vi "ScaleSquat_Angle.vi"(8 "ArmLength":cluster{"Upper":dbl, "Lower":dbl}, 9 "ScalingCoef Knee (1)":dbl=1.0, 10 "ScalingCoef Hip (1)":dbl=1.0, 11 "AverageJointAngles":dbl[][](array[numeric])) -> (1 "ScaledJointAngles":dbl[][](array[numeric]), 2 "ScaledGait":dbl[][](array[numeric]))   [LabVIEW 2016]
uses:
  <vilib>/Analysis/baseanly.llb/Real A x B.vi
  <vilib>/imath/engines/lvmath2/RunTimeEngine/NodeEndStatement/NIMS_NodeEndStatement_Output.vi
  <instcachedir>/0/NIMS_NodeEndStatement_Output_53EC0D466D134D7ABD903AC30B43404B.lvgen/NIMS_NodeEndStatement_Output_53EC0D466D134D7ABD903AC30B43404B_002.vi
  <vilib>/imath/engines/lvmath2/RunTimeEngine/ErrorHandling/NIMS_Finalize Error.vi
  <vilib>/Analysis/NI_AALBase.lvlib
panel:
  out "Waveform Graph 2":dbl[][](graph)
  out "JointAngles":dbl[][](graph)
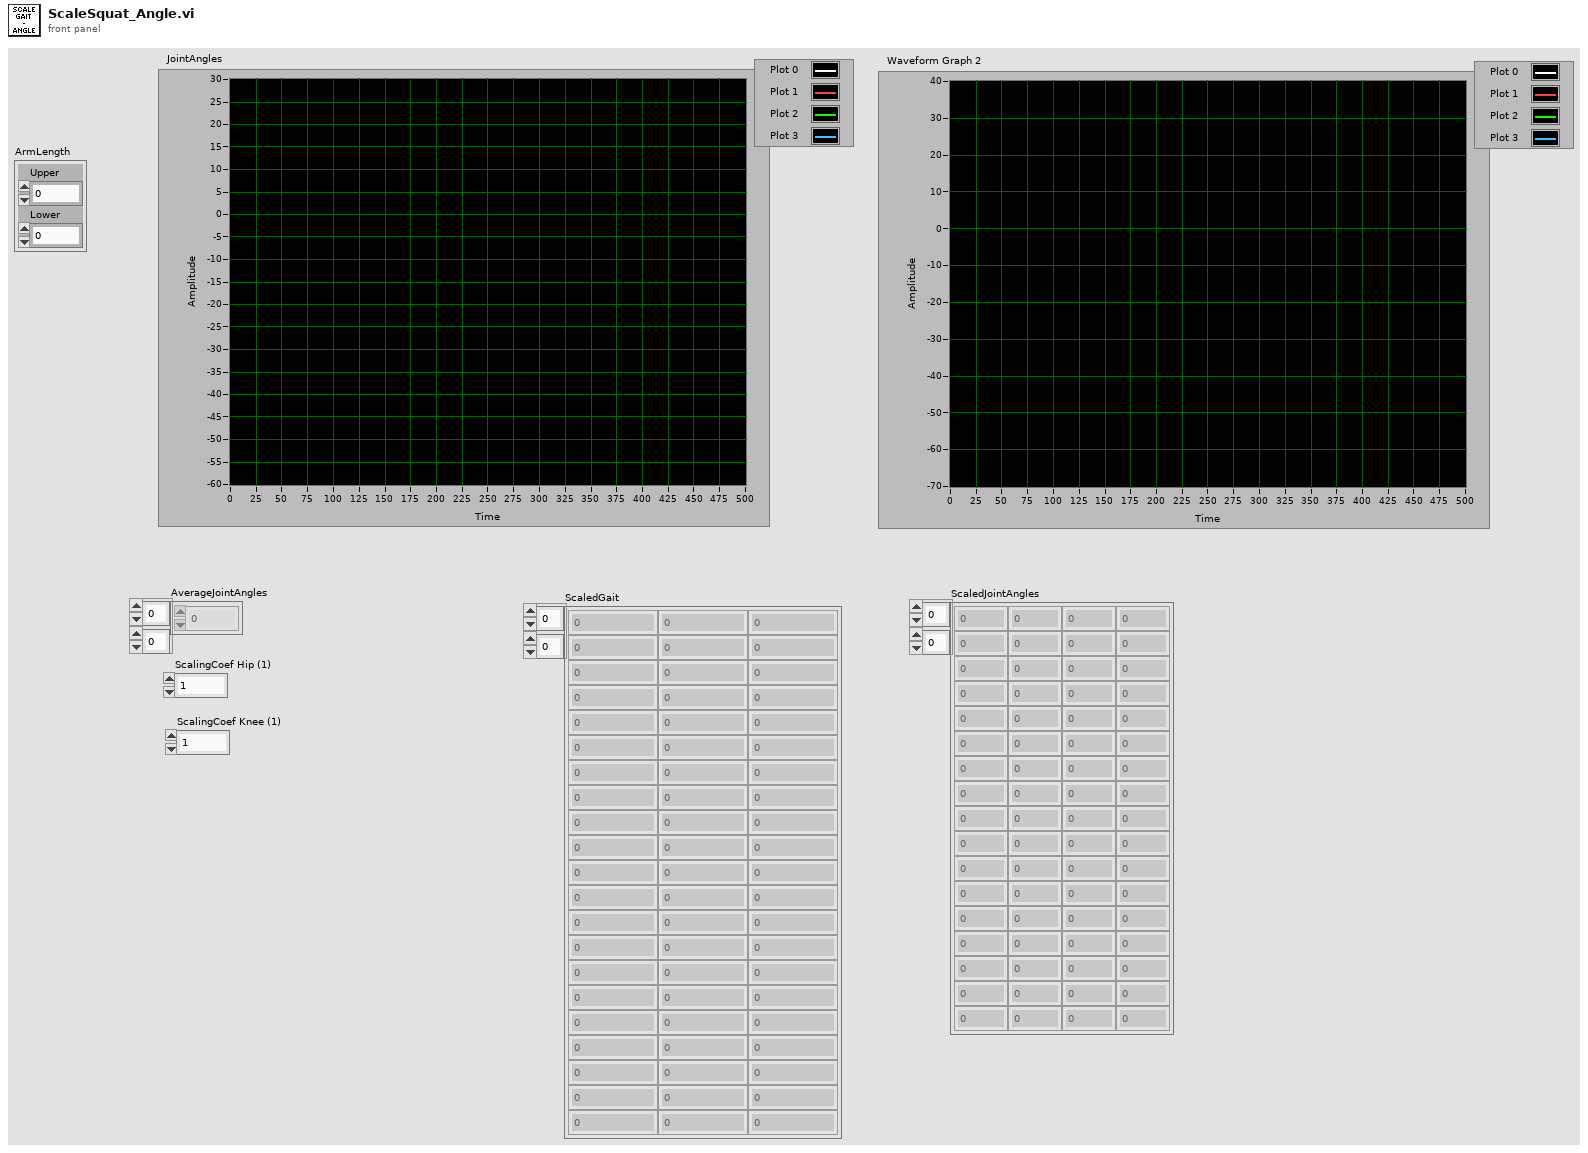
[diagram p1: front panel]
types:
  T1 = typedef "NI_Matrix.lvlib/RealMatrix.ctl" = dbl[][]
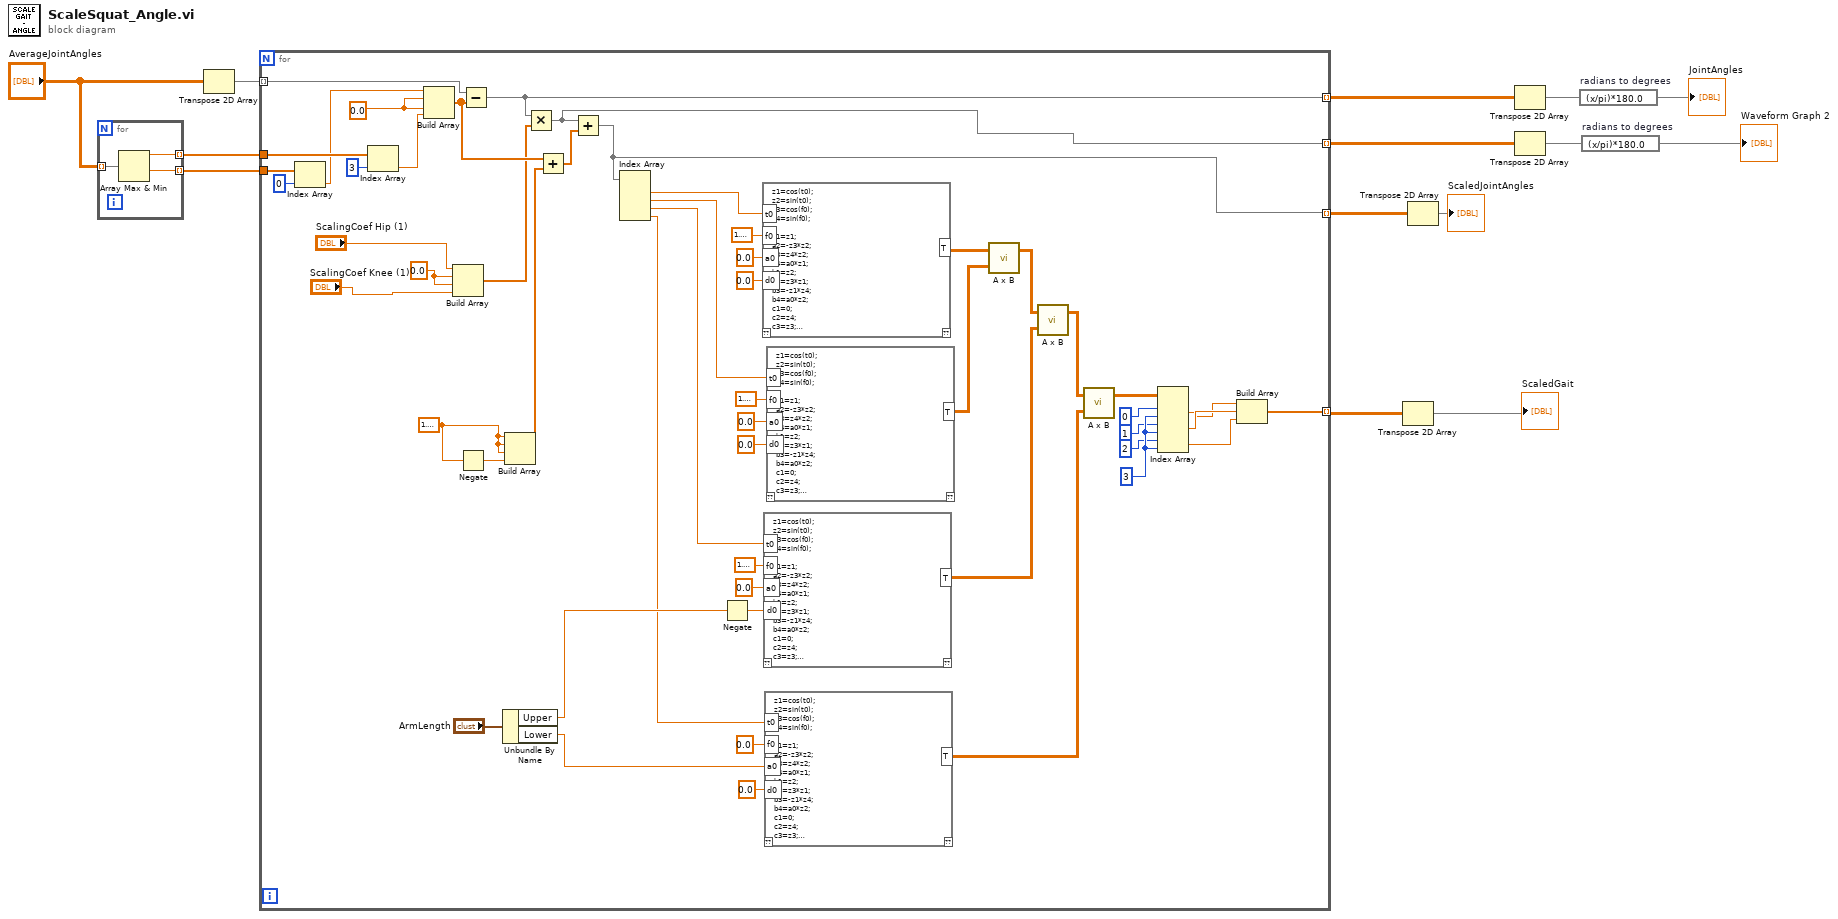
[diagram p0: block diagram]
diagram:
  n1 = for {
    tunnel: "AverageJointAngles" -> [w17] mode=indexing
    tunnel: [w16] -> w9 mode=indexing
    tunnel: [w15] -> w7 mode=indexing
    n2 = Array Max & Min(array=w17) -> (max value=w15:dbl, min value=w16:dbl)  [unwired: 2 out]
  }
  n3 = Transpose 2D Array(2D array="AverageJointAngles") -> (transposed array=w12:dbl[][])
  n4 = for {
    tunnel: w12 -> [w70] mode=indexing
    tunnel: [w65] -> w13 mode=indexing
    tunnel: w9 -> [w67]
    tunnel: [w29] -> w8 mode=indexing
    tunnel: w7 -> [w69]
    tunnel: [w41] -> w4 mode=indexing
    tunnel: [w28] -> w2 mode=indexing
    w19 = 0.0 ("element")
    w27 = 0.0 ("element")
    w22 = 1.5707963267948966
    w40 = 3 ("index (row)")
    n5 = Index Array(array=w67, index=0) -> (element=w66:dbl)
    n6 = Index Array(array=w69, index=3) -> (element=w30:dbl)
    n7 = Build Array(w66, w27, w27, w30) -> (w26:dbl[])
    n8 = Build Array("ScalingCoef Hip (1)", w19, w19, "ScalingCoef Knee (1)") -> (w21:dbl[])
    n9 = Negate(x=w22) -> (-x=w23:dbl)
    n10 = Subtract(x=w70, y=w26) -> (x-y=w65:dbl[])
    n11 = Unbundle By Name("ArmLength") -> ("Upper"=w35:dbl, "Lower"=w34:dbl)
    n12 = Build Array(w22, w22, w22, w23) -> (w24:dbl[])
    n13 = Multiply(x=w65, y=w21) -> (x*y=w29:dbl[])
    n14 = Add(x=w26, y=w24) -> (x+y=w25:dbl[])
    n15 = Add(x=w29, y=w25) -> (x+y=w28:dbl[])
    n16 = Index Array(array=w28) -> (element #1=w33:dbl, element #2=w60:dbl, element #3=w59:dbl, element #4=w32:dbl)  [unwired: 4 in]
    n17 = Negate(x=w35) -> (-x=w53:dbl)
    n18 = mathscript code="z1=cos(t0);\nz2=sin(t0);\nz3=cos(f0);\nz4=sin(f0);\n\na1=z1;\na2=-z3*z2;\na3=z4*z2;\na4=a0*z1;\nb1=z2;\nb2=z3*z1;\nb3=-z1*z4;\nb4=a0*z2;\nc1=0;\nc2=z4;\nc3=z3;\nc4=d0;\nd1=0;\nd2=0;\nd3=0;\nd4=1;\n\nT=[a1,a2,a3,a4;b1,b2,b3,b4;c1,c2,c3,c4;d1,d2,d3,d4];"("t0"=w33, "f0"=1.5707963267948966, "a0"=0.0, "d0"=0.0) -> ("T"=w51:dbl[][])  [unwired: 1 in, 1 out]
    n19 = mathscript code="z1=cos(t0);\nz2=sin(t0);\nz3=cos(f0);\nz4=sin(f0);\n\na1=z1;\na2=-z3*z2;\na3=z4*z2;\na4=a0*z1;\nb1=z2;\nb2=z3*z1;\nb3=-z1*z4;\nb4=a0*z2;\nc1=0;\nc2=z4;\nc3=z3;\nc4=d0;\nd1=0;\nd2=0;\nd3=0;\nd4=1;\n\nT=[a1,a2,a3,a4;b1,b2,b3,b4;c1,c2,c3,c4;d1,d2,d3,d4];"("t0"=w59, "f0"=1.5707963267948966, "a0"=0.0, "d0"=w53) -> ("T"=w48:dbl[][])  [unwired: 1 in, 1 out]
    n20 = mathscript code="z1=cos(t0);\nz2=sin(t0);\nz3=cos(f0);\nz4=sin(f0);\n\na1=z1;\na2=-z3*z2;\na3=z4*z2;\na4=a0*z1;\nb1=z2;\nb2=z3*z1;\nb3=-z1*z4;\nb4=a0*z2;\nc1=0;\nc2=z4;\nc3=z3;\nc4=d0;\nd1=0;\nd2=0;\nd3=0;\nd4=1;\n\nT=[a1,a2,a3,a4;b1,b2,b3,b4;c1,c2,c3,c4;d1,d2,d3,d4];"("t0"=w32, "f0"=0.0 ("a0"), "a0"=w34, "d0"=0.0) -> ("T"=w46:dbl[][])  [unwired: 1 in, 1 out]
    n21 = mathscript code="z1=cos(t0);\nz2=sin(t0);\nz3=cos(f0);\nz4=sin(f0);\n\na1=z1;\na2=-z3*z2;\na3=z4*z2;\na4=a0*z1;\nb1=z2;\nb2=z3*z1;\nb3=-z1*z4;\nb4=a0*z2;\nc1=0;\nc2=z4;\nc3=z3;\nc4=d0;\nd1=0;\nd2=0;\nd3=0;\nd4=1;\n\nT=[a1,a2,a3,a4;b1,b2,b3,b4;c1,c2,c3,c4;d1,d2,d3,d4];"("t0"=w60, "f0"=1.5707963267948966, "a0"=0.0, "d0"=0.0) -> ("T"=w50:dbl[][])  [unwired: 1 in, 1 out]
    n22 = call-poly <vilib>:"A x B.vi"("B"=w50, "A"=w51) -> ("A x B"=w49:T1)  [unwired: 1 out]
    n23 = call-poly <vilib>:"A x B.vi"("B"=w48, "A"=w49) -> ("A x B"=w47:T1)  [unwired: 1 out]
    n24 = call-poly <vilib>:"A x B.vi"("B"=w46, "A"=w47) -> ("A x B"=w45:T1)  [unwired: 1 out]
    n25 = Index Array(array=w45, index (row) #1=0 ("disabled index (col)"), index (col) #1=w40, index (row) #2=1 ("index (row)"), index (col) #2=w40, index (row) #3=2 ("index (row)"), index (col) #3=w40) -> (element #1=w42:dbl, element #2=w43:dbl, element #3=w44:dbl)
    n26 = Build Array(w42, w43, w44) -> (w41:dbl[])
  }
  n27 = Transpose 2D Array(2D array=w4) -> (transposed array=→"ScaledGait":dbl[][])
  n28 = Transpose 2D Array(2D array=w2) -> (transposed array=→"ScaledJointAngles":dbl[][])
  n29 = Transpose 2D Array(2D array=w13) -> (transposed array=w11:dbl[][])
  n30 = Transpose 2D Array(2D array=w8) -> (transposed array=w6:dbl[][])
  n31 = expression code="(x/pi)*180.0" "radians to degrees"(w11) -> (→"JointAngles":dbl[][])
  n32 = expression code="(x/pi)*180.0" "radians to degrees"(w6) -> (→"Waveform Graph 2":dbl[][])
